vi "cRIOModuleInfo.vi"(8 "error in (no error)":errorcluster, 9 "session":refnum<k21>="localhost", 10 "number of slots":i32, 11 "cRIO Backplane":T1) -> (0 "error out":errorcluster, 2 "cRIO Modules":T1[](array[typedef]))   [LabVIEW 2017, in "cRIODetectHW.lvlib"]
doc: "Gets information about cRIO modules, such as module ID, vendor name, model name, and serial number."
uses:
  <vilib>/addons/cRIODetectHW/cRIODetectHW.lvlib
  <vilib>/addons/cRIODetectHW/control/cRIO Product Info.ctl
  <vilib>/addons/cRIODetectHW/control/FPGARef.ctl
  <vilib>/nisyscfg/Close (Hardware).vi
  <vilib>/Utility/error.llb/Error Cluster From Error Code.vi
  <vilib>/rvi/errors/niLvFpgaAdjustHostInterfaceError.vi
  <vilib>/FPGAPlugInAG/Dynamic/niLvFpga_Close_Dynamic.vi
  <vilib>/rvi/interface/nirviReadWriteControl/nirviReadWriteControl.xnode
  <vilib>/rvi/interface/nirviCloseFPGA/nirviCloseFPGA.xnode
  NiFpgaLv.dll
  <vilib>/rvi/interface/Simulation/niFpgaSimulationCallBeginRW.vi
  <vilib>/nisyscfg/nisyscfg.lvlib
  <resource>/objmgr/nicontrollersysapi.rc
  <vilib>/addons/InsightCM/Devices/Shared/Cms/DAQmx/TSNcDAQ_AI.lvlib
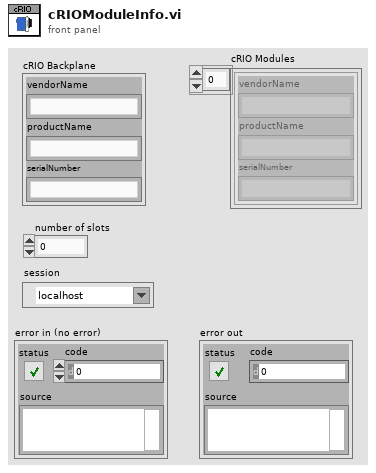
[diagram p1: front panel]
types:
  T1 = typedef "cRIODetectHW.lvlib/cRIO Product Info.ctl" = cluster{"vendorName":string, "productName":string, "serialNumber":string}
  T2 = typedef "cRIODetectHW.lvlib/FPGARef.ctl" = refnum<k20>
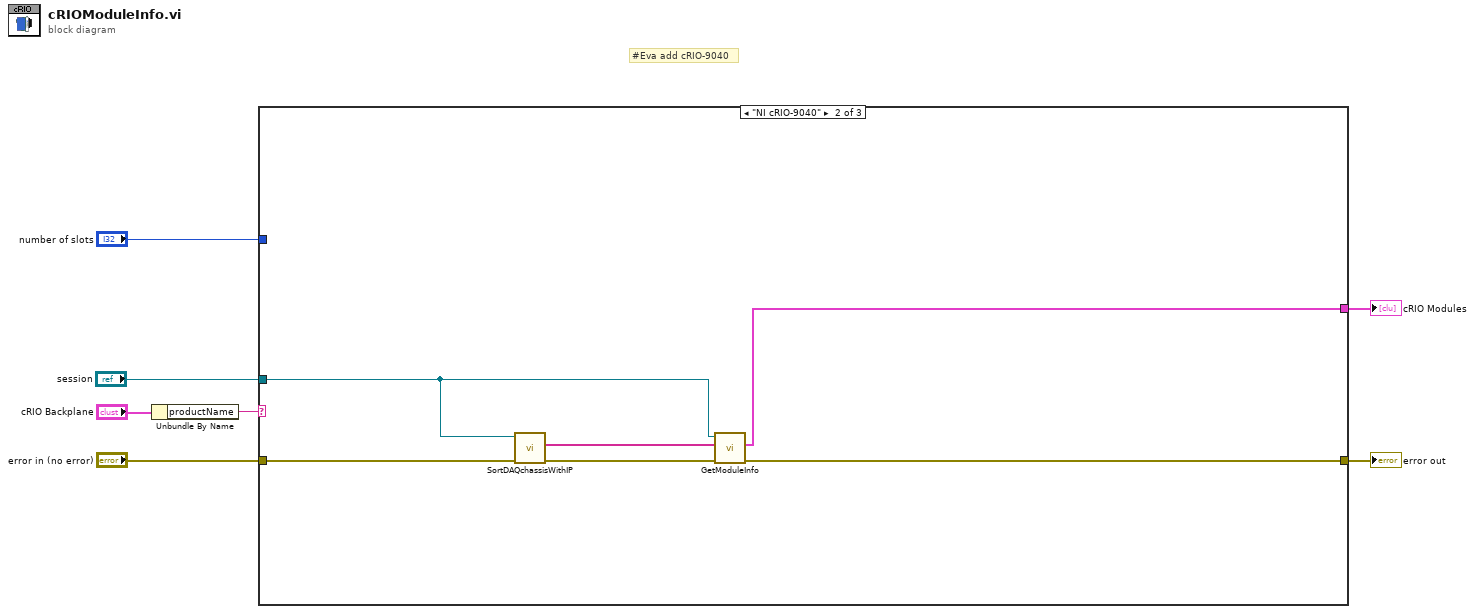
[diagram p0: block diagram]
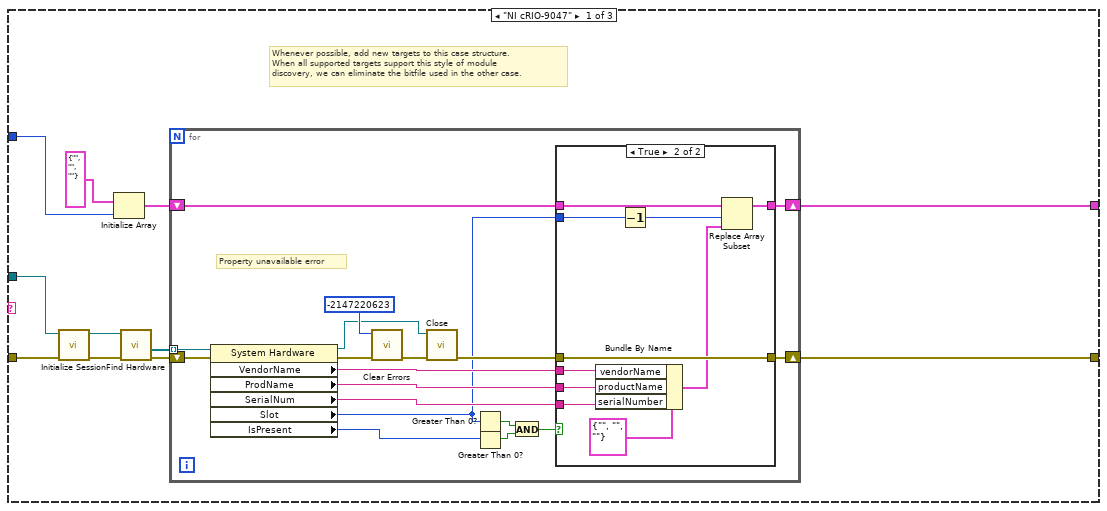
[diagram p2: hidden frame]
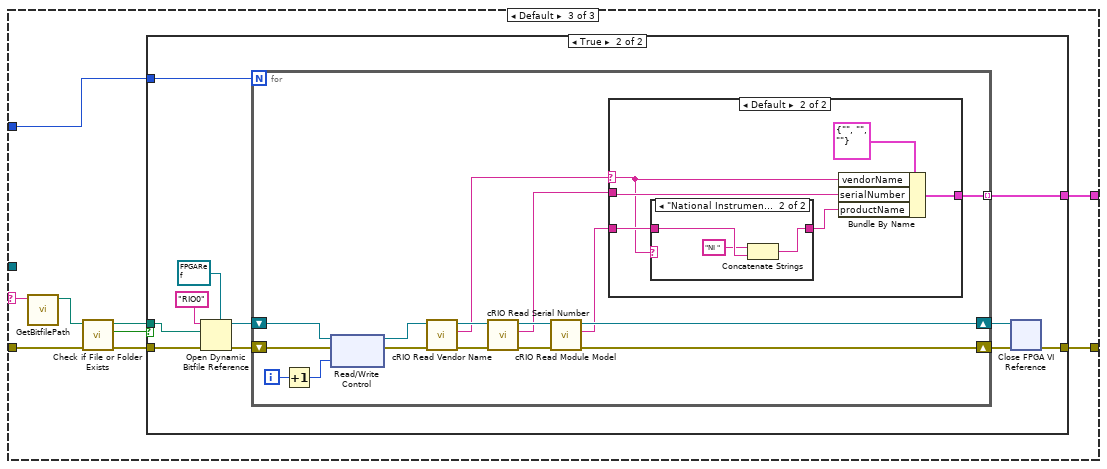
[diagram p4: hidden frame]
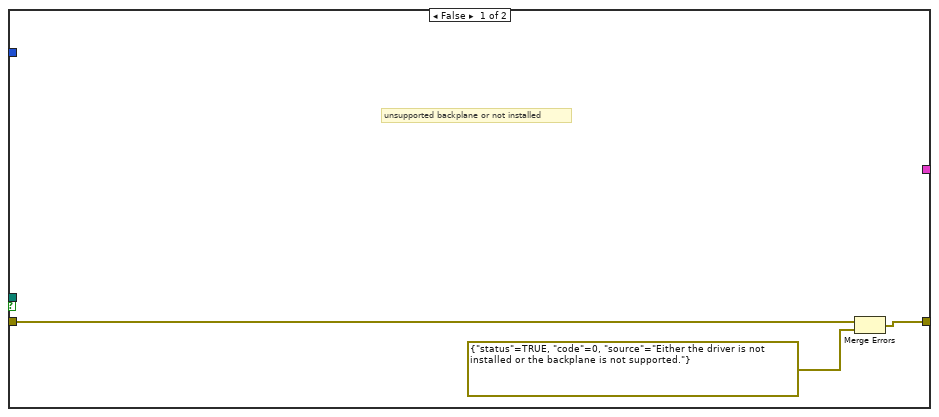
[diagram p5: hidden frame]
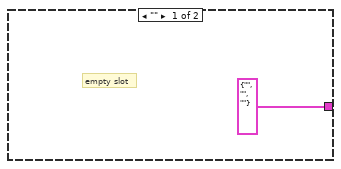
[diagram p6: hidden frame]
diagram:
  # "#Eva add cRIO-9040"
  n1 = Unbundle By Name("cRIO Backplane") -> ("productName"=w2:string)
  n2 = case shown="\"NI cRIO-9040\"" w2 {
    selector: w2 -> [_ _ w55]
    tunnel: [w8 w50 w63] -> w7
    tunnel: "number of slots" -> [w11 _ w62]
    tunnel: "error in (no error)" -> [w15 w54 w61]
    tunnel: [w9 w49 w56] -> w4
    tunnel: "session" -> [w16 w52 _]
    frame "NI cRIO-9047" {
      # "Whenever possible, add new targets to this case structure.\nWhen all supported targets support this style of module\ndiscovery, we can eliminate the bitfile used in the other case."
      n3 = call <vilib>:"Initialize Session.vi"("error in (no error)"=w15, "Target (localhost)"=w16) -> ("error out"=w17:errorcluster, "Session out"=w18:refnum<k21>)  [unwired: 8 in]
      n4 = Initialize Array(T1 {"vendorName"="", "productName"="", "serialNumber"=""} ("cRIO Module Info"), w11) -> (w10:T1[])
      n5 = call <vilib>:"Find Hardware.vi"("error in (no error)"=w17, "Session in"=w18) -> ("error out"=w14:errorcluster, "Resources out"=w13:refnum<k20>[])  [unwired: 6 in, 2 out]
      n6 = for {
        shift-right: [w23] -> w8
        shift-left: w14 -> [w36]
        tunnel: w13 -> [w35] mode=indexing
        shift-right: [w22] -> w9
        shift-left: w10 -> [w21]
        # "Property unavailable error"
        n7 = property class="System Hardware"(reference=w35, error in=w36) -> (reference out=w19:refnum<k20>, error out=w33:errorcluster, "VendorName"=w26:string, "ProdName"=w25:string, "SerialNum"=w24:string, "Slot"=w20:i32, "IsPresent"=w30:i32)
        n8 = call <vilib>:"Clear Errors.vi"("error in (no error)"=w33, "specific error code to clear (0: all)"=-2147220623) -> ("error out"=w32:errorcluster)  [unwired: 4 in, 1 out]
        n9 = call-poly <vilib>:"Close.vi"("error in (no error)"=w32, "Resource in"=w19) -> ("error out"=w31:errorcluster)  [unwired: 9 in]
        n10 = Greater Than 0?(x=w20) -> (x > 0?=w28:bool)
        n11 = Greater Than 0?(x=w30) -> (x > 0?=w29:bool)
        n12 = And(x=w28, y=w29) -> (x .and. y?=w27:bool)
        n13 = case shown="True" w27 {
          tunnel: w31 -> [w38 w44]
          tunnel: w26 -> [_ w47]
          tunnel: w25 -> [_ w46]
          tunnel: w24 -> [_ w45]
          tunnel: [w38 w44] -> w23
          tunnel: [w37 w42] -> w22
          tunnel: w21 -> [w37 w43]
          tunnel: w20 -> [_ w39]
          frame False {
          }
          frame True {
            n14 = Bundle By Name(cluster=T1 {"vendorName"="", "productName"="", "serialNumber"=""} ("cRIO Module Info"), "vendorName"=w47, "productName"=w46, "serialNumber"=w45) -> (w41:T1)
            n15 = Decrement(x=w39) -> (x-1=w40:i32)
            n16 = Replace Array Subset(array=w43, new element=w41, index=w40) -> (w42:T1[])
          }
        }
      }
    }
    frame "NI cRIO-9040" {
      n17 = call <vilib>:"SortDAQchassisWithIP.vi"("error in (no error)"=w54, "Target (localhost)"=w52) -> ("error out"=w51:errorcluster, "SN Number"=w53:string[])  [unwired: 8 in]
      n18 = call <vilib>:"GetModuleInfo.vi"("error in (no error)"=w51, "SN Number"=w53, "Target (localhost)"=w52) -> ("error out"=w50:errorcluster, "Modules"=w49:T1[])  [unwired: 7 in]
    }
    frame Default {
      n19 = call <vilib>:"GetBitfilePath.vi"("productName"=w55) -> ("bitfile path"=w60:path)  [unwired: 10 in]
      n20 = call <vilib>:"Check if File or Folder Exists.vi"("error in (no error)"=w61, "path"=w60) -> ("error out"=w59:errorcluster, "file or folder exists?"=w57:bool, "dup path"=w58:path)  [unwired: 7 in]
      n21 = case shown="True" w57 {
        tunnel: [w66 w76] -> w63
        tunnel: [_ w75] -> w56
        tunnel: w62 -> [_ w74]
        tunnel: w59 -> [w64 w73]
        tunnel: w58 -> [_ w67]
        frame False {
          # "unsupported backplane or not installed"
          n22 = Merge Errors(w64, errorcluster {"status"=TRUE, "code"=0, "source"="Either the driver is not installed or the backplane is not supported."} ("error out")) -> (w66:errorcluster)
        }
        frame True {
          n23 = Open Dynamic Bitfile Reference(0:"RIO0" ("Device address"), 1:w67, 3:w73, 4:T2 refnum ("FPGA VI Reference")) -> (5:w72:T2, 8:w71:errorcluster)  [unwired: 1 in]
          n24 = for {
            N: w74 -> [_]
            tunnel: [w84] -> w75 mode=indexing
            shift-right: [w92] -> w70
            shift-left: w71 -> [w81]
            shift-right: [w93] -> w77
            shift-left: w72 -> [w80]
            i -> [w79]
            n25 = Increment(x=w79) -> (x+1=w78:i32)
            n26 = xnode "Read/Write Control"("FPGA VI Reference In"=w80, "error in"=w81, "Module"=w78) -> ("FPGA VI Reference Out"=w86:T2, "error out"=w87:errorcluster)
            n27 = call <vilib>:"cRIO Read Vendor Name.vi"("error in (no error)"=w87, "Refnum in"=w86) -> ("error out"=w88:errorcluster, "Vendor Name"=w83:string, "Refnum out"=w89:T2)  [unwired: 7 in]
            n28 = call <vilib>:"cRIO Read Serial Number.vi"("error in (no error)"=w88, "Refnum in"=w89) -> ("error out"=w91:errorcluster, "Serial Number"=w82:string, "Refnum out"=w90:T2)  [unwired: 7 in]
            n29 = call <vilib>:"cRIO Read Module Model.vi"("error in (no error)"=w91, "Refnum in"=w90) -> ("error out"=w92:errorcluster, "Module Model"=w85:string, "Refnum out"=w93:T2)  [unwired: 7 in]
            n30 = case shown="Default" w83 {
              selector: w83 -> [_ w95]
              tunnel: w85 -> [_ w98]
              tunnel: [T1 {"vendorName"="", "productName"="", "serialNumber"=""} ("cRIO Module Info") w100] -> w84
              tunnel: w82 -> [_ w96]
              frame "" {
                # "empty slot"
              }
              frame Default {
                n31 = case shown="\"National Instruments\"" w95 {
                  tunnel: w98 -> [w101 w104]
                  tunnel: [w101 w103] -> w97
                  frame Default {
                  }
                  frame "National Instruments" {
                    n32 = Concatenate Strings("NI " ("string"), w104) -> (w103:string)
                  }
                }
                n33 = Bundle By Name(cluster=T1 {"vendorName"="", "productName"="", "serialNumber"=""} ("cRIO Module Info"), "vendorName"=w95, "serialNumber"=w96, "productName"=w97) -> (w100:T1)
              }
            }
          }
          n34 = xnode "Close FPGA VI Reference"("FPGA VI Reference In"=w77, "error in"=w70) -> ("error out"=w76:errorcluster)
        }
      }
    }
  }
  "error out" <- w7
  "cRIO Modules" <- w4
